vi "JoystickMove.vi"(7 "JogSpeed":dbl[](array[numeric]), 8 "error in":errorcluster, 9 "Speed":dbl, 10 "Axis":i32, 11 "ESP300":refnum<visa-resource-name>) -> (0 "error out":errorcluster, 5 "JogSpeed":dbl[](array[numeric]))   [LabVIEW 2012, in "ESP300.lvlib"]
uses:
  ESP300.lvlib
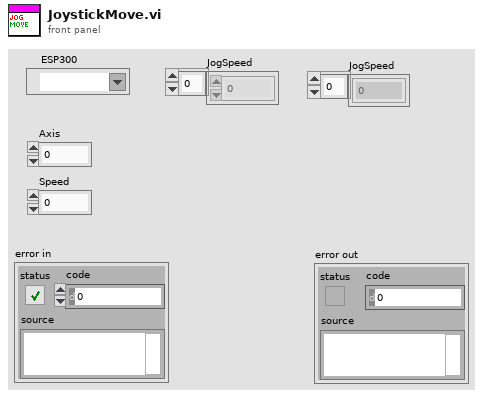
[diagram p1: front panel]
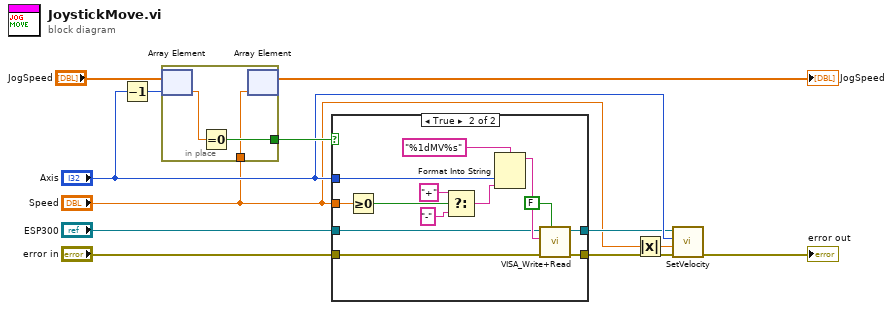
[diagram p0: block diagram]
diagram:
  n1 = Decrement(x="Axis") -> (x-1=w8:i32)
  n2 = in-place {
    in-place-border: [w14] -> w7
    in-place-border: "Speed" -> [w13]
    n3 = in-place-array #1("JogSpeed", w8) -> (w15:dbl)
    n4 = Equal To 0?(x=w15) -> (x = 0?=w14:bool)
    n5 = in-place-array #1(w13) -> (→"JogSpeed":dbl[])  [unwired: 1 out]
  }
  n6 = case shown="True" w7 {
    tunnel: [w16 w28] -> w6
    tunnel: "error in" -> [w16 w27]
    tunnel: "Axis" -> [_ w26]
    tunnel: "Speed" -> [_ w22]
    tunnel: [w17 w24] -> w4
    tunnel: "ESP300" -> [w17 w23]
    frame False {
    }
    frame True {
      n7 = Greater Or Equal To 0?(x=w22) -> (x >= 0?=w18:bool)
      n8 = Select(t="+", s=w18, f="-") -> (s? t:f=w21:string)
      n9 = Format Into String(format string="%1dMV%s", w26, w21) -> (resulting string=w29:string)  [unwired: 2 in, 1 out]
      n10 = call "VISA_Write+Read.vi"("Read?(T)"=FALSE ("Read?"), "error in (no error)"=w27, "Write Buffer"=w29, "VISA resource name"=w23) -> ("error out"=w28:errorcluster, "VISA resource name out"=w24:refnum<visa-resource-name>)  [unwired: 5 in, 1 out]
    }
  }
  n11 = Absolute Value(x="Speed") -> (abs(x)=w2:dbl)
  n12 = call "SetVelocity.vi"("error in"=w6, "Velocity"=w2, "Axial #"="Axis", "VISA resource"=w4) -> ("error out"=→"error out":errorcluster)  [unwired: 7 in]
